vi "Close AuroraTracker.vi"(8 "Error In":errorcluster, 11 "OptiTrack Data":T1) -> (0 "Error Out":errorcluster)   [LabVIEW 2017]
uses:
  Controls/Tracking Data Multi Body.ctl
  Controls/Packet Data.ctl
  Controls/Rigid Body Info.ctl
  Controls/Position.ctl
  Controls/Orientation.ctl
  Controls/Tracker Type.ctl
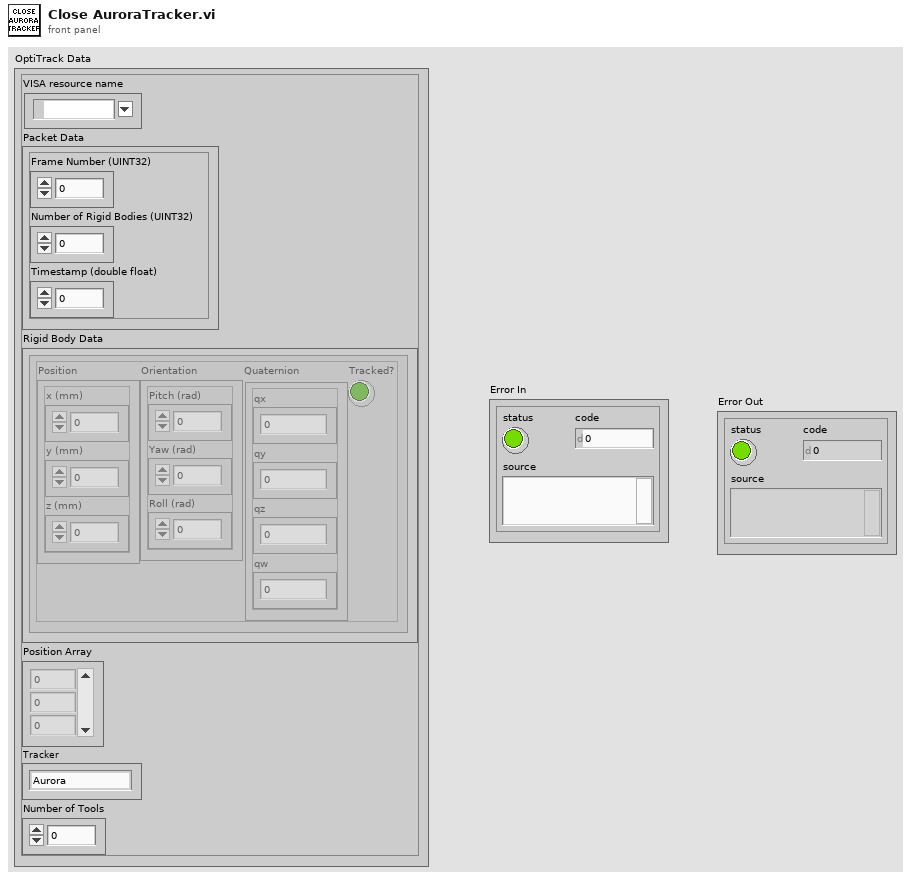
[diagram p1: front panel]
types:
  T1 = typedef "Tracking Data Multi Body.ctl" = cluster{"VISA resource name":refnum<visa-resource-name>, "Packet Data":T2, "Rigid Body Data":T3[], "Position Array":dbl[][], "Tracker":T6, "Number of Tools":u32}
  T2 = typedef "Packet Data.ctl" = cluster{"Frame Number (UINT32)":u32, "Number of Rigid Bodies (UINT32)":u32, "Timestamp (double float)":dbl}
  T3 = typedef "Rigid Body Info.ctl" = cluster{"Position":T4, "Orientation":T5, "Quaternion":cluster{"qx":sgl, "qy":sgl, "qz":sgl, "qw":sgl}, "Tracked?":bool}
  T4 = typedef "Position.ctl" = cluster{"x (mm)":sgl, "y (mm)":sgl, "z (mm)":sgl}
  T5 = typedef "Orientation.ctl" = cluster{"Pitch (rad)":sgl, "Yaw (rad)":sgl, "Roll (rad)":sgl}
  T6 = typedef "Tracker Type.ctl" = enum16{"Aurora", "OptiTrack"}
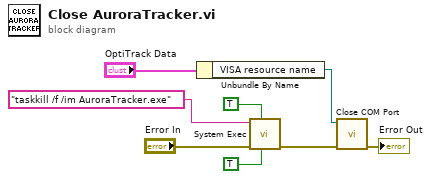
[diagram p0: block diagram]
diagram:
  n1 = Unbundle By Name("OptiTrack Data") -> ("VISA resource name"=w3:refnum<visa-resource-name>)
  n2 = call <vilib>:"System Exec.vi"("run minimized? (F)"=TRUE, "wait until completion? (T)"=TRUE, "error in (no error)"="Error In", "command line"="taskkill /f /im AuroraTracker.exe" ("String")) -> ("error out"=w2:errorcluster)  [unwired: 4 in, 3 out]
  n3 = call "Close COM Port.vi"("error in (no error)"=w2, "VISA Refnum in"=w3) -> ("error out"=→"Error Out":errorcluster)  [unwired: 9 in]
